vi "get_FPGA_reference.vi"(8 "error in (no error)":errorcluster) -> (0 "error out":errorcluster, 1 "is empty?":bool, 2 "FPGA VI Reference":T1)   [LabVIEW 2010, in "FPGAWrapperRK110512Fiber_Spiral.lvclass"]
uses:
  FPGAWrapperRK110512Fiber_Spiral.lvclass
  FPGA_VI_Reference.ctl
  class_data.vi
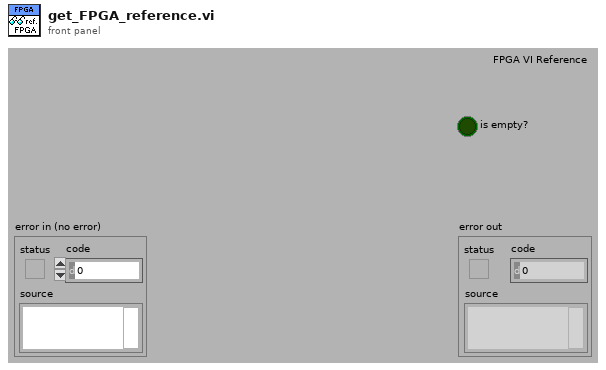
[diagram p1: front panel]
types:
  T1 = typedef "FPGAWrapperRK110512Fiber_Spiral.lvclass/FPGA_VI_Reference.ctl" = refnum<k20>
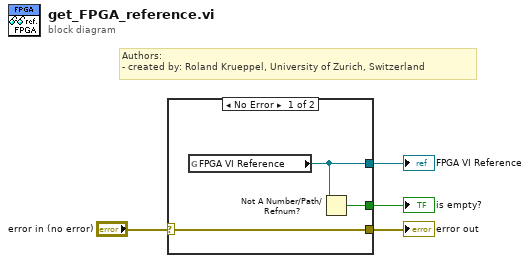
[diagram p0: block diagram]
diagram:
  # "Authors: \n- created by: Roland Krueppel, University of Zurich, Switzerland"
  n1 = case shown="No Error" "error in (no error)" {
    selector: "error in (no error)" -> [w7 w8]
    tunnel: [w7 w8] -> w3
    tunnel: [w6 _] -> w2
    tunnel: [w5 _] -> w1
    frame No Error {
      n2 = global read "class_data.vi" "FPGA VI Reference"() -> (w6:T1)
      n3 = Not A Number/Path/Refnum?(number/path/refnum=w6) -> (NaN/Path/Refnum?=w5:bool)
    }
    frame Error {
    }
  }
  "error out" <- w3
  "FPGA VI Reference" <- w2
  "is empty?" <- w1
